vi "Set Connection Properties.vi"(8 "error in (no error)":errorcluster, 10 "AutoSelect":T2, 11 "Device Item Ref in":T1 format="%.0x") -> (0 "error out":errorcluster, 3 "Item Ref out":T1 format="%.0x")   [LabVIEW 2017, in "Chassis TimeSync System Explorer.lvlib"]
uses:
  Chassis TimeSync System Explorer.lvlib
  Shared/Connection Settings.ctl
  Shared/Mode.ctl
  Shared/External Pin.ctl
  Shared/Routes.ctl
  Shared/Route.ctl
  <vilib>/NI Veristand/Custom Device API/Custom Device Item Ref.ctl
  Shared/Constants.vi
  <vilib>/NI Veristand/Custom Device API/Set Item Property (U16).vi
  <vilib>/NI Veristand/Custom Device API/Set Item Property (Boolean).vi
  Shared/Chassis TimeSync Shared.lvlib
  <vilib>/NI Veristand/Custom Device API/Custom Device API.lvlib
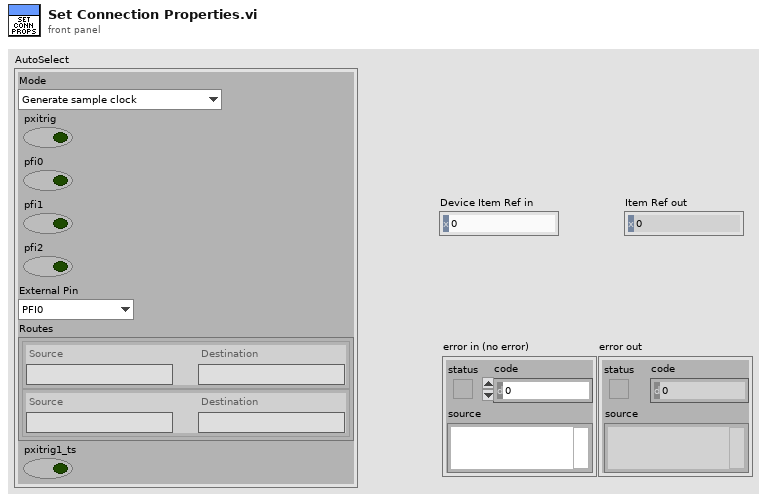
[diagram p1: front panel]
types:
  T1 = typedef "Custom Device API.lvlib/Custom Device Item Ref.ctl" = u64
  T2 = typedef "Chassis TimeSync Shared.lvlib/Connection Settings.ctl" = cluster{"Mode":T3, "pxitrig":bool, "pfi0":bool, "pfi1":bool, "pfi2":bool, "External Pin":T4, "Routes":T5, "pxitrig1_ts":bool}
  T3 = typedef "Chassis TimeSync Shared.lvlib/Mode.ctl" = enum16{"Generate sample clock", "Route sample clock out of chassis", "Route sample clock into chassis", "Custom routes"}
  T4 = typedef "Chassis TimeSync Shared.lvlib/External Pin.ctl" = enum16{"PFI0", "PFI1", "PFI2"}
  T5 = typedef "Chassis TimeSync Shared.lvlib/Routes.ctl" = T6[]
  T6 = typedef "Chassis TimeSync Shared.lvlib/Route.ctl" = cluster{"Source":string, "Destination":string}
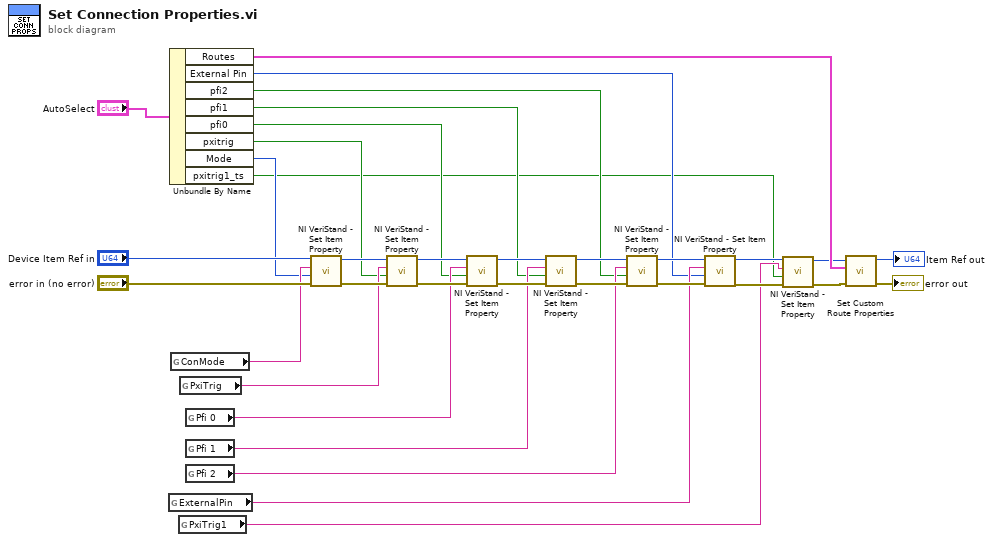
[diagram p0: block diagram]
diagram:
  n1 = global read "Constants.vi" "ExternalPin"() -> (w17:string)
  n2 = Unbundle By Name("AutoSelect") -> ("Routes"=w9:T5, "External Pin"=w8:T4, "pfi2"=w10:bool, "pfi1"=w11:bool, "pfi0"=w12:bool, "pxitrig"=w13:bool, "Mode"=w7:T3, "pxitrig1_ts"=w3:bool)
  n3 = global read "Constants.vi" "ConMode"() -> (w32:string)
  n4 = global read "Constants.vi" "PxiTrig1"() -> (w4:string)
  n5 = global read "Constants.vi" "PxiTrig"() -> (w29:string)
  n6 = global read "Constants.vi" "Pfi 0"() -> (w26:string)
  n7 = global read "Constants.vi" "Pfi 1"() -> (w23:string)
  n8 = global read "Constants.vi" "Pfi 2"() -> (w20:string)
  n9 = call-poly <vilib>:"NI VeriStand - Set Item Property.vi"("error in (no error)"="error in (no error)", "Value"=w7, "Property Name"=w32, "Item Ref in"="Device Item Ref in") -> ("error out"=w30:errorcluster, "Item Ref out"=w31:T1)  [unwired: 5 in, 1 out]
  n10 = call-poly <vilib>:"NI VeriStand - Set Item Property.vi"("error in (no error)"=w30, "Value"=w13, "Property Name"=w29, "Item Ref in"=w31) -> ("error out"=w27:errorcluster, "Item Ref out"=w28:T1)  [unwired: 5 in, 1 out]
  n11 = call-poly <vilib>:"NI VeriStand - Set Item Property.vi"("error in (no error)"=w27, "Value"=w12, "Property Name"=w26, "Item Ref in"=w28) -> ("error out"=w24:errorcluster, "Item Ref out"=w25:T1)  [unwired: 5 in, 1 out]
  n12 = call-poly <vilib>:"NI VeriStand - Set Item Property.vi"("error in (no error)"=w24, "Value"=w11, "Property Name"=w23, "Item Ref in"=w25) -> ("error out"=w21:errorcluster, "Item Ref out"=w22:T1)  [unwired: 5 in, 1 out]
  n13 = call-poly <vilib>:"NI VeriStand - Set Item Property.vi"("error in (no error)"=w21, "Value"=w10, "Property Name"=w20, "Item Ref in"=w22) -> ("error out"=w19:errorcluster, "Item Ref out"=w18:T1)  [unwired: 5 in, 1 out]
  n14 = call-poly <vilib>:"NI VeriStand - Set Item Property.vi"("error in (no error)"=w19, "Value"=w8, "Property Name"=w17, "Item Ref in"=w18) -> ("error out"=w5:errorcluster, "Item Ref out"=w6:T1)  [unwired: 5 in, 1 out]
  n15 = call-poly <vilib>:"NI VeriStand - Set Item Property.vi"("error in (no error)"=w5, "Value"=w3, "Property Name"=w4, "Item Ref in"=w6) -> ("error out"=w2:errorcluster, "Item Ref out"=w1:T1)  [unwired: 5 in, 1 out]
  n16 = call "Set Custom Route Properties.vi"("error in (no error)"=w2, "Routes"=w9, "Item Ref in"=w1) -> ("error out"=→"error out":errorcluster, "Item Ref out"=→"Item Ref out":T1)  [unwired: 7 in]
